vi "Initialize VIs Stream.vi"(8 "error in (no error)":errorcluster, 11 "Channel in":refnum<class "Channel.lvclass">) -> (0 "error out":errorcluster, 3 "Channel out":refnum<class "Channel.lvclass">)   [LabVIEW 2018, in "Channel.lvclass"]
uses:
  Channel.lvclass
  Channel.lvclass/Channel.ctl
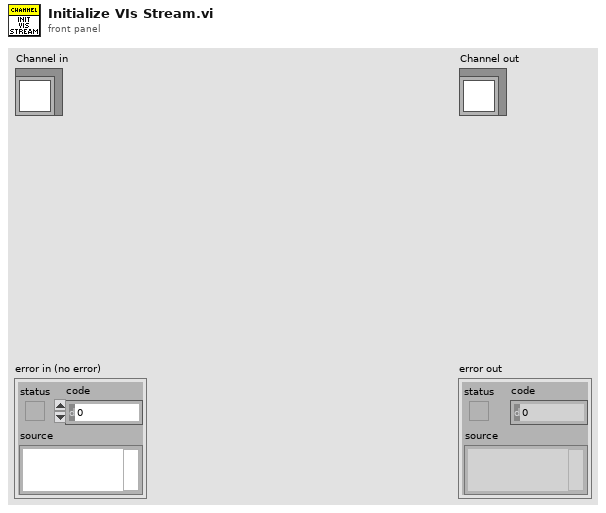
[diagram p1: front panel]
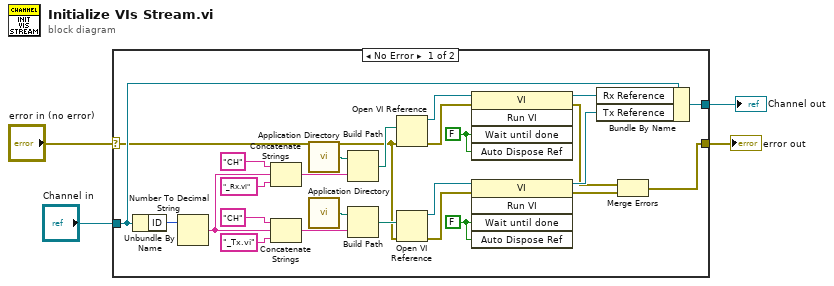
[diagram p0: block diagram]
diagram:
  n1 = case shown="No Error" "error in (no error)" {
    selector: "error in (no error)" -> [w6 w32]
    tunnel: [w9 w32] -> w3
    tunnel: [w22 w31] -> w1
    tunnel: "Channel in" -> [w23 w31]
    frame No Error {
      w17 = FALSE ("Wait Until Done")
      w27 = FALSE ("Wait Until Done")
      n2 = Unbundle By Name(w23) -> ("ID"=w5:u8)
      n3 = Number To Decimal String(number=w5) -> (decimal integer string=w13:string)  [unwired: 1 in]
      n4 = Concatenate Strings("CH" ("name or relative path"), w13, "_Rx.vi" ("name or relative path")) -> (w24:string)
      n5 = Concatenate Strings("CH" ("name or relative path"), w13, "_Tx.vi" ("name or relative path")) -> (w20:string)
      n6 = call <vilib>:"Application Directory.vi"() -> ("Application Directory"=w30:path)
      n7 = call <vilib>:"Application Directory.vi"() -> ("Application Directory"=w14:path)
      n8 = Build Path(base path=w30, name or relative path=w24) -> (appended path=w29:path)
      n9 = Build Path(base path=w14, name or relative path=w20) -> (appended path=w15:path)
      n10 = Open VI Reference(vi path=w29, error in (no error)=w6) -> (vi reference=w28:refnum<vi>, error out=w8:errorcluster)  [unwired: 4 in]
      n11 = Open VI Reference(vi path=w15, error in (no error)=w6) -> (vi reference=w16:refnum<vi>, error out=w7:errorcluster)  [unwired: 4 in]
      n12 = invoke class="VI" method="Run VI"(reference=w28, error in=w8, "Wait until done"=w27, "Auto Dispose Ref"=w27) -> (reference out=w21:refnum<vi>, error out=w10:errorcluster)  [unwired: 1 in, 3 out]
      n13 = invoke class="VI" method="Run VI"(reference=w16, error in=w7, "Wait until done"=w17, "Auto Dispose Ref"=w17) -> (reference out=w12:refnum<vi>, error out=w11:errorcluster)  [unwired: 1 in, 3 out]
      n14 = Bundle By Name(cluster=w23, "Rx Reference"=w21, "Tx Reference"=w12) -> (w22:refnum<class "Channel.lvclass">)
      n15 = Merge Errors(w10, w11) -> (w9:errorcluster)
    }
    frame Error {
    }
  }
  "error out" <- w3
  "Channel out" <- w1
